vi "DriveConversionSensorUnits.vi"() -> (3 "Inches per Sensor Units":dbl=0.03726)   [LabVIEW 2018]
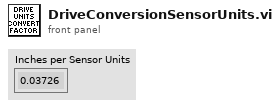
[diagram p1: front panel]
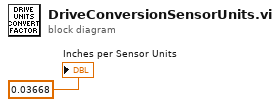
[diagram p0: block diagram]
diagram:
  "Inches per Sensor Units" <- 0.03668 ("Sensor Units to Inches")
